vi "Add Notification to Map.vi"(7 "Alias":string, 8 "error in (no error)":errorcluster, 9 "Value":T1, 10 "Symbol Name":string, 11 "TwinCAT ADS in":refnum<class "TwinCAT ADS.lvclass">) -> (0 "error out":errorcluster, 2 "Success?":bool, 3 "TwinCAT ADS out":refnum<class "TwinCAT ADS.lvclass">)   [LabVIEW 2018, in "TwinCAT ADS.lvclass"]
uses:
  TwinCAT ADS.lvclass
  Controls/Notifcation Map Value.ctl
  TwinCAT ADS.lvclass/TwinCAT ADS.ctl
  <vilib>/Utility/error.llb/Trim Whitespace.vi
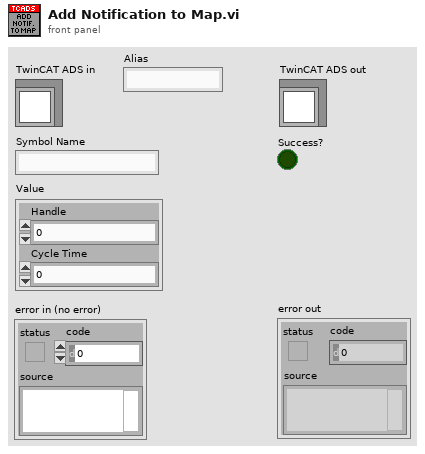
[diagram p1: front panel]
types:
  T1 = typedef "TwinCAT ADS.lvclass/Notifcation Map Value.ctl" = cluster{"Handle":i32, "Cycle Time":i32}
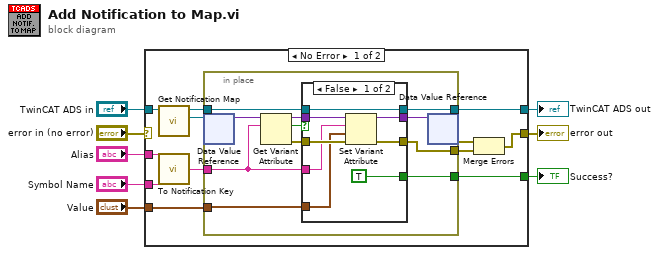
[diagram p0: block diagram]
diagram:
  n1 = case shown="No Error" "error in (no error)" {
    selector: "error in (no error)" -> [_ w43]
    tunnel: "TwinCAT ADS in" -> [w19 w44]
    tunnel: "Value" -> [w20 _]
    tunnel: "Symbol Name" -> [w10 _]
    tunnel: [w16 w44] -> w6
    tunnel: [w13 w43] -> w5
    tunnel: [w12 _] -> w2
    tunnel: "Alias" -> [w11 _]
    frame No Error {
      n2 = call "Get Notification Map.vi"("TwinCAT ADS in"=w19) -> ("Notification Map"=w18:refnum<data-value>, "TwinCAT ADS out"=w17:refnum<class "TwinCAT ADS.lvclass">)  [unwired: 8 in, 1 out]
      n3 = call "To Notification Key.vi"("Alias"=w11, "Symbol Name"=w10) -> ("Key"=w9:string)  [unwired: 5 in]
      n4 = in-place {
        in-place-border: w20 -> [w27]
        in-place-border: w9 -> [w26]
        in-place-border: w17 -> [w24]
        in-place-border: [w23] -> w16
        in-place-border: [w22] -> w14
        in-place-border: [w21] -> w12
        n5 = in-place-dvr #1(w18) -> (w31:variant)  [unwired: 1 out]
        n6 = Get Variant Attribute(Variant=w31, name=w26) -> (duplicate Variant=w30:variant, found=w25:bool, error out=w28:errorcluster)  [unwired: 2 in, 1 out]
        n7 = case shown="False" w25 {
          tunnel: w30 -> [w39 w42]
          tunnel: [w38 w42] -> w29
          tunnel: w28 -> [w37 w40]
          tunnel: w27 -> [w35 _]
          tunnel: w26 -> [w36 _]
          tunnel: w24 -> [w34 w41]
          tunnel: [w34 w41] -> w23
          tunnel: [w33 w40] -> w22
          tunnel: [TRUE _] -> w21
          frame False {
            n8 = Set Variant Attribute(Variant=w39, name=w36, value=w35, error in=w37) -> (Variant out=w38:variant, error out=w33:errorcluster)  [unwired: 1 out]
          }
          frame True {
          }
        }
        n9 = in-place-dvr #1(w29) -> (w15:errorcluster)  [unwired: 1 out]
      }
      n10 = Merge Errors(w15, w14) -> (w13:errorcluster)
    }
    frame Error {
    }
  }
  "error out" <- w5
  "TwinCAT ADS out" <- w6
  "Success?" <- w2
